vi "get UI reference.vi"(8 "error in":errorcluster, 11 "execution settings in":refnum<class "execution settings.lvclass">) -> (0 "error out":errorcluster, 2 "VI Refnum":refnum<vi>, 3 "execution settings out":refnum<class "execution settings.lvclass">)   [LabVIEW 2013, in "execution settings.lvclass"]
uses:
  execution settings.lvclass
  exec ui.vi
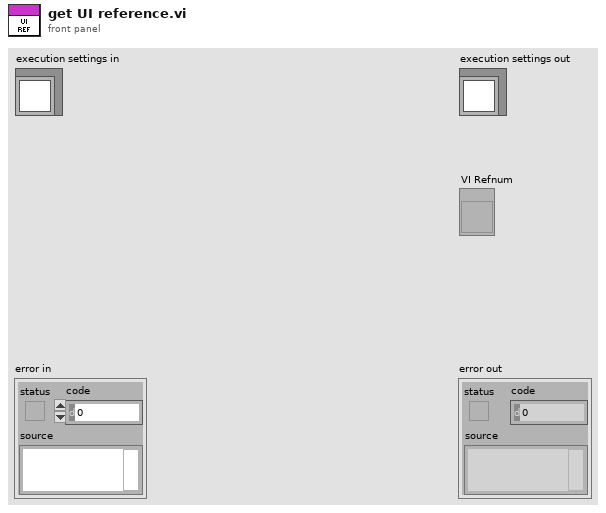
[diagram p1: front panel]
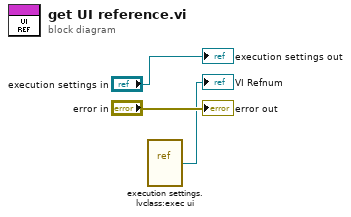
[diagram p0: block diagram]
diagram:
  n1 = vi-ref "execution settings.lvclass:exec ui.vi"() -> (→"VI Refnum":refnum<vi>)
  "error out" <- "error in"
  "execution settings out" <- "execution settings in"
